vi "Request Topic Actor by Name.vi"(8 "error in (no error)":errorcluster, 10 "Topic Actor":string, 11 "Topic Actor Look Up Table in":refnum<class "Topic Actor Look Up Table.lvclass">) -> (0 "error out":errorcluster, 1 "Found?":bool, 2 "Topic Actor Descriptor":refnum<class "Topic Actor Descriptor.lvclass">, 3 "Topic Actor Look Up Table out":refnum<class "Topic Actor Look Up Table.lvclass">)   [LabVIEW 2016, in "Stream Mediator.lvlib" / "Topic Actor Look Up Table.lvclass"]
doc: "--\nCopyright © 2017 Composed SystemsI All rights reserved.\n\nAuthor: Jon McBee <jon.mcbee@composed.io>\n\nThis library is provided \"AS IS\" ,WITHOUT WARRANTIES OR\nCONDITIONS OF ANY KIND, either express or implied.\n\nComposed Systems -- composed.io\n\nStream 0.0.1.1\nJon McBee - Composed Systems\nCopyright (c) 2017, Composed Systems"
uses:
  <userlib>/Composed Systems/Stream/Mediator/Classes/Topic Actor Look Up Table/Topic Actor Look Up Table.lvclass
  C:/Program Files (x86)/National Instruments/LabVIEW 2016/user.lib/Composed Systems/Stream/Look Up Table/Look Up Table/Look Up Table.lvclass
  <userlib>/Composed Systems/Stream/Mediator/Classes/Topic Actor Descriptor/Topic Actor Descriptor.lvclass
  <userlib>/Composed Systems/Stream/Look Up Table/Look Up Table/Look Up Table.lvclass
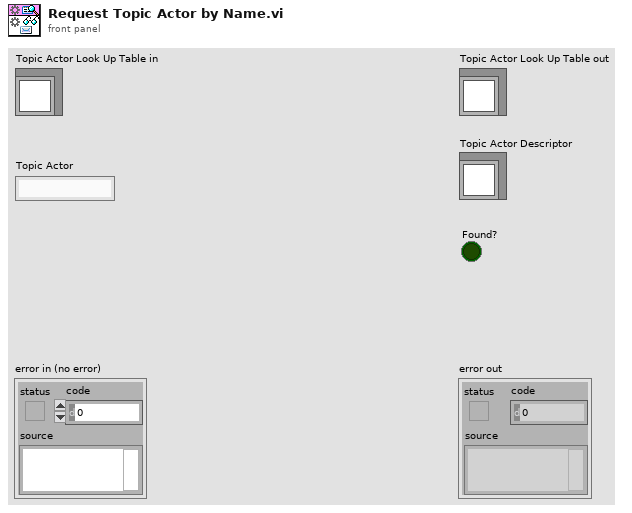
[diagram p1: front panel]
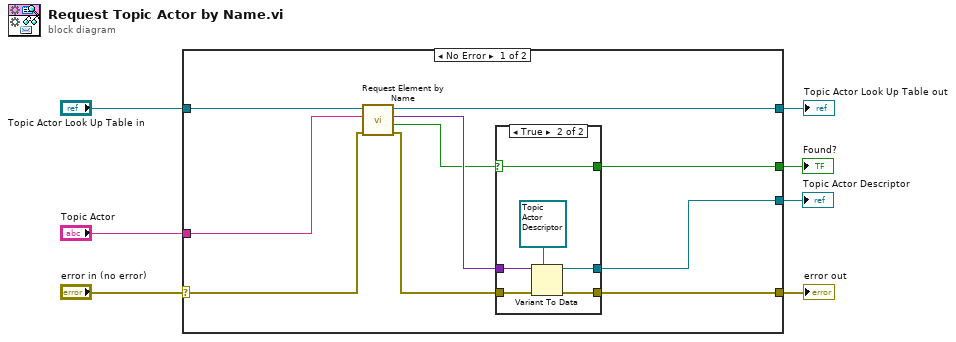
[diagram p0: block diagram]
diagram:
  n1 = case shown="No Error" "error in (no error)" {
    selector: "error in (no error)" -> [w12 w27]
    tunnel: [w17 w27] -> w6
    tunnel: [w11 w26] -> w4
    tunnel: "Topic Actor Look Up Table in" -> [w14 w26]
    tunnel: "Topic Actor" -> [w13 _]
    tunnel: [w15 _] -> w1
    tunnel: [w16 _] -> w2
    frame No Error {
      n2 = call <userlib>:"Request Element by Name.vi"("error in (no error)"=w12, "Name"=w13, "Look Up Table in"=w14) -> ("error out"=w8:errorcluster, "Found?"=w9:bool, "Element"=w10:variant, "Look Up Table out"=w11:refnum<class "Topic Actor Look Up Table.lvclass">)  [unwired: 5 in]
      n3 = case shown="True" w9 {
        selector: w9 -> [w19 w20]
        tunnel: w10 -> [_ w25]
        tunnel: w8 -> [w18 w24]
        tunnel: [w18 w23] -> w17
        tunnel: [_ w22] -> w16
        tunnel: [w19 w20] -> w15
        frame False {
        }
        frame True {
          n4 = Variant To Data(error in=w24, type=refnum<class "Topic Actor Descriptor.lvclass"> refnum ("Topic Actor Descriptor"), Variant=w25) -> (data=w22:refnum<class "Topic Actor Descriptor.lvclass">, error out=w23:errorcluster)
        }
      }
    }
    frame Error {
    }
  }
  "error out" <- w6
  "Topic Actor Look Up Table out" <- w4
  "Topic Actor Descriptor" <- w2
  "Found?" <- w1
